vi "Command Loop.vi"(8 "Error in":errorcluster, 10 "Queue Refs":variant, 11 "Device Reference in":T1 format="%.0x") -> ()   [LabVIEW 2026, in "Nominal Core Streaming Engine.lvlib"]
uses:
  <vilib>/NI VeriStand/Custom Device API/Custom Device Item Ref.ctl
  <vilib>/NI VeriStand/Custom Device API/Message Response (String).ctl
  <vilib>/NI VeriStand/Custom Device API/Message Response (Byte Array).ctl
  Nominal Core Streaming Engine.lvlib
  <vilib>/NI VeriStand/Custom Device API/Custom Device API.lvlib
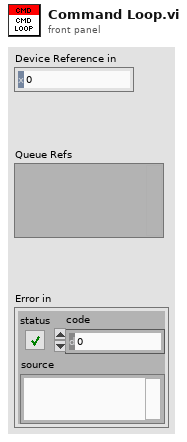
[diagram p1: front panel]
types:
  T1 = typedef "Custom Device API.lvlib/Custom Device Item Ref.ctl" = u64
  T2 = typedef "Custom Device API.lvlib/Custom Device Engine Event Ref.ctl" = refnum<event-registration>
  T3 = typedef "Custom Device API.lvlib/Message Response (String).ctl" = cluster{"Response":string, "Error":errorcluster}
  T4 = typedef "Custom Device API.lvlib/Message Response (Byte Array).ctl" = cluster{"Response":u8[], "Error":errorcluster}
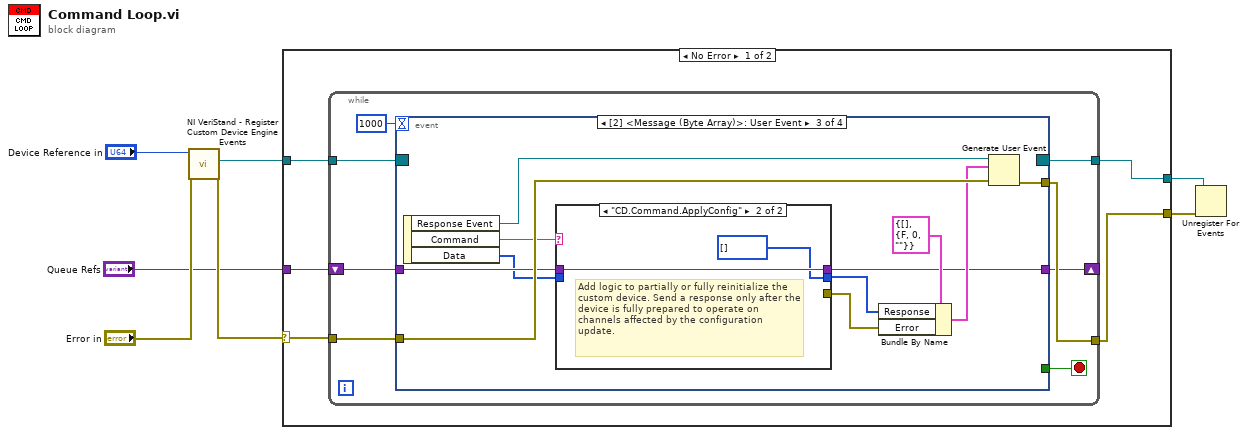
[diagram p0: block diagram]
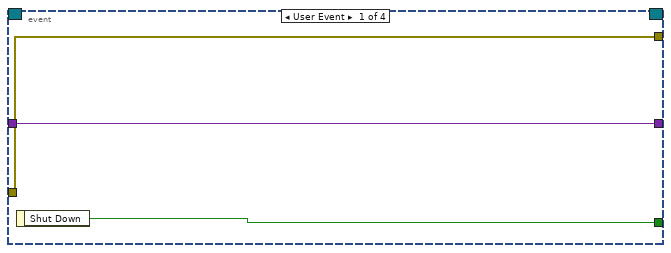
[diagram p2: hidden frame]
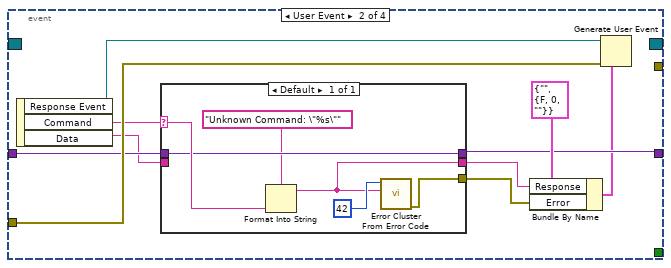
[diagram p3: hidden frame]
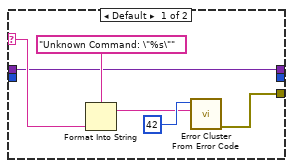
[diagram p4: hidden frame]
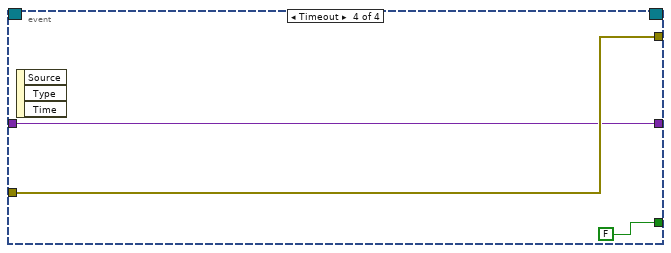
[diagram p5: hidden frame]
diagram:
  n1 = call <vilib>:"NI VeriStand - Register Custom Device Engine Events.vi"("error in (no error)"="Error in", "Device Ref in"="Device Reference in") -> ("error out"=w5:errorcluster, "Custom Device Engine Event Ref"=w2:T2)  [unwired: 7 in, 1 out]
  n2 = case shown="No Error" w5 {
    selector: w5 -> [w12 w62]
    tunnel: [w10 _] -> w4
    tunnel: [w11 w62] -> w7
    tunnel: w2 -> [w9 _]
    tunnel: "Queue Refs" -> [w8 _]
    frame No Error {
      n3 = while {
        tunnel: [w17] -> w10
        tunnel: w9 -> [w16]
        shift-right: [w13] -> _
        shift-left: w8 -> [w14]
        tunnel: w12 -> [w20]
        tunnel: [w19] -> w11
        stop <- w18 stop-if-true
        n4 = event shown="[2] <Message (Byte Array)>: User Event" {
          selector: w16 -> [_ _ _ _]
          dyn-events: [_ _ _ _] -> w17
          timeout: 1000 -> [_ _ _ _]
          tunnel: [w22 _ _ FALSE ("Shut Down")] -> w18
          tunnel: [w23 _ w48 w61] -> w19
          tunnel: w20 -> [w23 w33 w49 w61]
          tunnel: w14 -> [w21 w28 w42 w59]
          tunnel: [w21 w27 w41 w59] -> w13
          event User Event {
            n5 = event-data() -> ("Shut Down"=w22:bool)  [unwired: 1 in]
          }
          event User Event {
            n6 = event-data() -> ("Response Event"=w29:refnum<user-event>, "Command"=w30:string, "Data"=w26:string)  [unwired: 1 in]
            n7 = case shown="Default" w30 {
              selector: w30 -> [w37]
              tunnel: w28 -> [w36]
              tunnel: [w36] -> w27
              tunnel: w26 -> [_]
              tunnel: [w34] -> w24
              tunnel: [w39] -> w32
              frame Default {
                n8 = Format Into String(format string="Unknown Command: \"%s\"", w37) -> (resulting string=w34:string)  [unwired: 2 in, 1 out]
                n9 = call <vilib>:"Error Cluster From Error Code.vi"("error message (\"\")"=w34, "error code (0)"=42) -> ("error out"=w39:errorcluster)  [unwired: 7 in]
              }
            }
            n10 = Bundle By Name(cluster=T3 {"Response"="", "Error"={"status"=FALSE, "code"=0, "source"=""}} ("event data"), "Response"=w24, "Error"=w32) -> (w25:T3)
            n11 = Generate User Event(user event=w29, event data cluster=w25, error in=w33) -> ()  [unwired: 1 in, 2 out]
          }
          event User Event {
            n12 = event-data() -> ("Response Event"=w47:refnum<user-event>, "Command"=w43:string, "Data"=w40:u8[])  [unwired: 1 in]
            n13 = case shown="\"CD.Command.ApplyConfig\"" w43 {
              selector: w43 -> [w53 _]
              tunnel: [w56 _] -> w50
              tunnel: [_ u8[] [] ("unsigned byte array")] -> w45
              tunnel: w42 -> [w51 w58]
              tunnel: [w51 w58] -> w41
              tunnel: w40 -> [_ _]
              frame Default {
                n14 = Format Into String(format string="Unknown Command: \"%s\"", w53) -> (resulting string=w52:string)  [unwired: 2 in, 1 out]
                n15 = call <vilib>:"Error Cluster From Error Code.vi"("error message (\"\")"=w52, "error code (0)"=42) -> ("error out"=w56:errorcluster)  [unwired: 7 in]
              }
              frame "CD.Command.ApplyConfig" {
                # "Add logic to partially or fully reinitialize the custom device. Send a response only after the device is fully prepared to operate on channels affected by the configuration update."
              }
            }
            n16 = Bundle By Name(cluster=T4 {"Response"=[], "Error"={"status"=FALSE, "code"=0, "source"=""}} ("event data"), "Response"=w45, "Error"=w50) -> (w44:T4)
            n17 = Generate User Event(user event=w47, event data cluster=w44, error in=w49) -> (error out=w48:errorcluster)  [unwired: 1 in, 1 out]
          }
          event Timeout {
            n18 = event-data() -> ()  [unwired: 1 in, 3 out]
          }
        }
      }
    }
    frame Error {
    }
  }
  n19 = Unregister For Events(event registration refnum=w4, error in=w7) -> ()  [unwired: 1 out]
